vi "Is Feature Enabled.vi"(6 "Force Read from DLL? (F)":bool, 8 "error in":errorcluster, 11 "Feature Name":string) -> (0 "error out":errorcluster, 3 "Feature Enabled?":bool)   [LabVIEW 2019, in "grpc-lvsupport.lvlib"]
uses:
  grpc-lvsupport.lvlib
  <vilib>/Utility/error.llb/Error Cluster From Error Code.vi
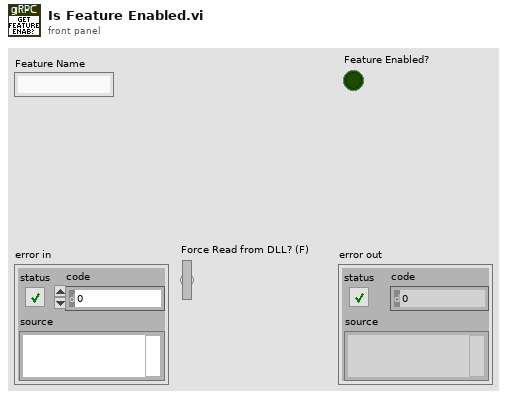
[diagram p1: front panel]
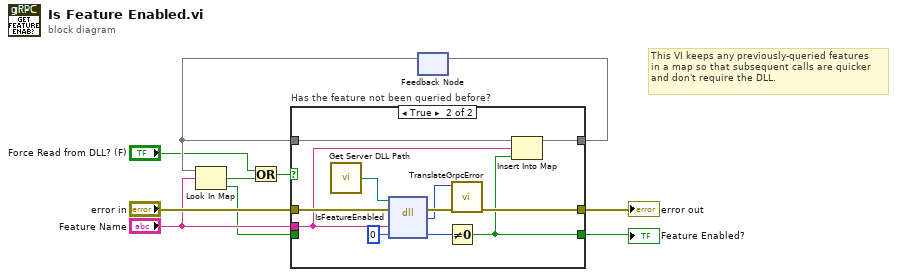
[diagram p0: block diagram]
diagram:
  # "This VI keeps any previously-queried features\nin a map so that subsequent calls are quicker\nand don't require the DLL."
  n1 = feedback #1() -> (w7:map{string, bool})  [unwired: 1 in]
  n2 = Look In Map(map=w7, key="Feature Name") -> (key not found?=w4:bool, value=w2:bool)  [unwired: 1 in]
  n3 = Or(x="Force Read from DLL? (F)", y=w4) -> (x .or. y?=w5:bool)
  n4 = case "Has the feature not been queried before?" shown="True" w5 {
    tunnel: "error in" -> [w12 w24]
    tunnel: [w12 w21] -> w9
    tunnel: "Feature Name" -> [_ w16]
    tunnel: w7 -> [w11 w17]
    tunnel: [w11 w15] -> w6
    tunnel: w2 -> [w13 _]
    tunnel: [w13 w14] -> w1
    frame False {
    }
    frame True {
      n5 = call "Get Server DLL Path.vi"() -> ("Server dll path"=w22:path)
      n6 = dll-call lib="?" fn="IsFeatureEnabled"(path in=w22, error in=w24, "featureName"=w16, "featureEnabled"=u8 0) -> (error out=w23:errorcluster, "return type"=w20:i32, "featureEnabled"=w18:u8)  [unwired: 2 in, 1 out]
      n7 = Not Equal To 0?(x=w18) -> (x != 0?=w14:bool)
      n8 = call "TranslateGrpcError.vi"("error in"=w23, "Error Code"=w20) -> ("error out"=w21:errorcluster)  [unwired: 9 in]
      n9 = Insert Into Map(map in=w17, key=w16, value=w14) -> (map out=w15:map{string, bool})  [unwired: 2 out]
    }
  }
  "error out" <- w9
  "Feature Enabled?" <- w1
  n10 = feedback-in #1(w6) -> ()
